vi "Pre Launch Init.vi"(11 "Simulated User Console Actor in":refnum<class "Simulated Display Console Actor.lvclass">) -> (0 "error out":errorcluster, 3 "Simulated User Console Actor out":refnum<class "Simulated Display Console Actor.lvclass">)   [LabVIEW 2019, in "Simulated Display Console Actor.lvlib" / "Simulated Display Console Actor.lvclass"]
doc: "(<B>Filename</B>: Actor Framework.lvlib:Actor.lvclass:Pre Launch Init.vi)\n\nDefines behavior that occurs after the Launch Nested Actor method is invoked but before the actor's Actor Core method begins running.\n\nBy default, this method does nothing. A descendant class may override it to define behavior."
uses:
  Simulated Display Console Actor.lvclass
  Simulated Display Console Actor.lvclass/Simulated Display Console Actor.ctl
  Display Console/Display Console/Display Console Actor.lvclass
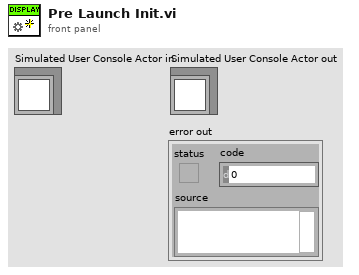
[diagram p1: front panel]
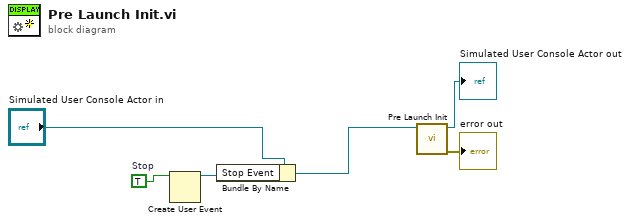
[diagram p0: block diagram]
diagram:
  w4 = TRUE  # Stop
  n1 = Create User Event(user event datatype=w4) -> (user event=w2:refnum<user-event>)  [unwired: 1 in, 1 out]
  n2 = Bundle By Name(cluster="Simulated User Console Actor in", "Stop Event"=w2) -> (w1:refnum<class "Simulated Display Console Actor.lvclass">)
  n3 = call-parent "Pre Launch Init.vi"("Actor in"=w1) -> ("error out"=→"error out":errorcluster, "Actor out"=→"Simulated User Console Actor out":refnum<class "Simulated Display Console Actor.lvclass">)  [unwired: 9 in]
